vi "Get Cells (2D Row Part String).vi"(6 "Column":i32, 8 "error in (no error)":errorcluster, 9 "Row":i32, 10 "Sheet Reference":refnum<k24>) -> (0 "error out":errorcluster, 2 "Sheet Reference out":refnum<k24>, 5 "Values":string[][](array[string]))   [LabVIEW 2014]
doc: "Reads a row from the Sheet Reference. Row specifies which row to read from. Column specifies the starting column to read from (default of 0 for the full row)."
uses:
  C:/Users/LENOVO/Desktop/CodeSpace GUI/LVExcel/Resources/NPOI 2.1.1 dotnet2/NPOI.dll
  Resources/NPOI 2.1.1 dotnet2/NPOI.dll
  <vilib>/ErrorRing/Error Ring.xnode
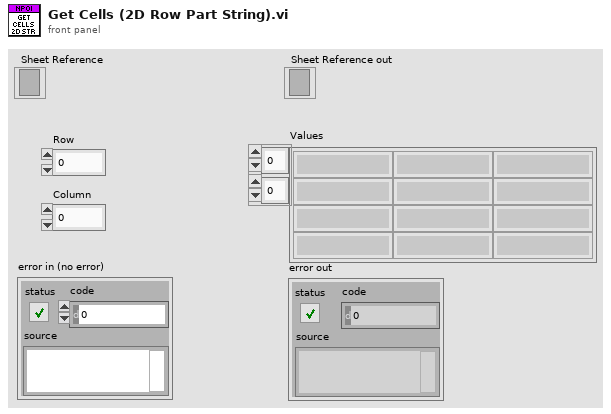
[diagram p1: front panel]
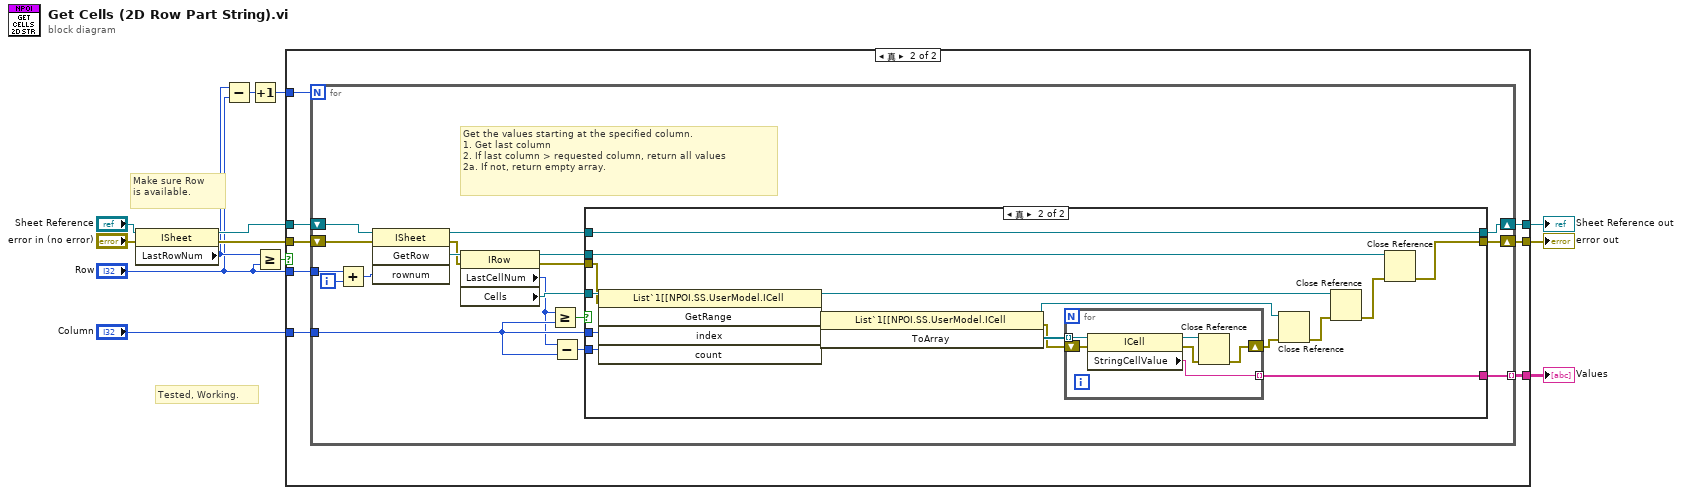
[diagram p0: block diagram]
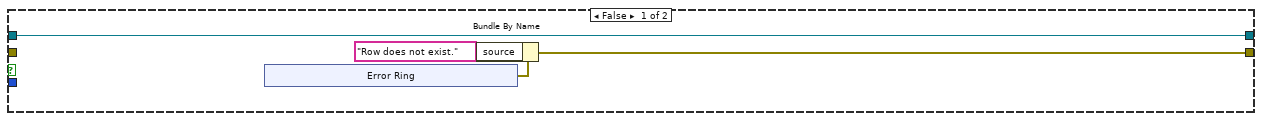
[diagram p2: hidden frame]
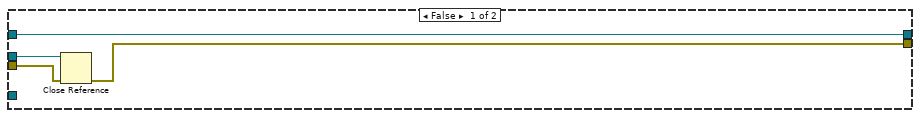
[diagram p3: hidden frame]
diagram:
  # "Tested, Working."
  # "Make sure Row\nis available."
  n1 = property class="ISheet"(reference="Sheet Reference", error in="error in (no error)") -> (reference out=w6:refnum<k24>, error out=w8:errorcluster, "LastRowNum"=w3:i32)
  n2 = Subtract(x=w3, y="Row") -> (x-y=w4:i32)
  n3 = Increment(x=w4) -> (x+1=w1:i32)
  n4 = Greater Or Equal?(x=w3, y="Row") -> (x >= y?=w5:bool)
  n5 = case shown="真" w5 {
    tunnel: w8 -> [_ w26]
    tunnel: w6 -> [w14 w25]
    tunnel: "Row" -> [_ w24]
    tunnel: [w14 w23] -> w13
    tunnel: [_ w22] -> w12
    tunnel: [w15 w21] -> w11
    tunnel: "Column" -> [_ w20]
    tunnel: w1 -> [_ w19]
    frame False {
      n6 = xnode "Error Ring"() -> ("错误输出"=w17:errorcluster)
      n7 = Bundle By Name(cluster=w17, "source"="Row does not exist.") -> (w15:errorcluster)
    }
    frame True {
      n8 = for {
        N: w19 -> [_]
        tunnel: w24 -> [w39]
        tunnel: [w37] -> w22 mode=indexing
        tunnel: w20 -> [w35]
        shift-right: [w38] -> w23
        shift-left: w25 -> [w40]
        shift-right: [w36] -> w21
        shift-left: w26 -> [w41]
        i -> [w27]
        # "Get the values starting at the specified column.\n1. Get last column\n2. If last column > requested column, return all values\n2a. If not, return empty array."
        n9 = Add(x=w39, y=w27) -> (x+y=w28:i32)
        n10 = invoke class="ISheet" method="GetRow"(reference=w40, error in=w41, "rownum"=w28) -> (reference out=w42:refnum<k24>, error out=w43:errorcluster, "GetRow"=w44:refnum<k24>)  [unwired: 1 in, 1 out]
        n11 = property class="IRow"(reference=w44, error in=w43) -> (reference out=w32:refnum<k24>, error out=w31:errorcluster, "LastCellNum"=w30:i16, "Cells"=w34:refnum<k24>)
        n12 = Greater Or Equal?(x=w30, y=w35) -> (x >= y?=w33:bool)
        n13 = Subtract(x=w30, y=w35) -> (x-y=w29:i32)
        n14 = case shown="真" w33 {
          tunnel: [_ w64] -> w37
          tunnel: w34 -> [_ w62]
          tunnel: w32 -> [w48 w54]
          tunnel: w31 -> [w47 w60]
          tunnel: [w46 w52] -> w36
          tunnel: w42 -> [w45 w51]
          tunnel: [w45 w51] -> w38
          tunnel: w35 -> [_ w50]
          tunnel: w29 -> [_ w49]
          frame False {
            n15 = Close Reference(reference=w48, error in (no error)=w47) -> (error out=w46:errorcluster)
          }
          frame True {
            n16 = invoke class="List`1[[NPOI.SS.UserModel.ICell" method="GetRange"(reference=w62, error in=w60, "index"=w50, "count"=w49) -> (reference out=w56:refnum<k24>, error out=w59:errorcluster, "GetRange"=w63:refnum<k24>)  [unwired: 1 in, 2 out]
            n17 = invoke class="List`1[[NPOI.SS.UserModel.ICell" method="ToArray"(reference=w63, error in=w59) -> (reference out=w58:refnum<k24>, error out=w61:errorcluster, "ToArray"=w65:refnum<k24>[])  [unwired: 1 in]
            n18 = for {
              tunnel: w65 -> [w71] mode=indexing
              tunnel: [w70] -> w64 mode=indexing
              shift-right: [w67] -> w57
              shift-left: w61 -> [w66]
              n19 = property class="ICell"(reference=w71, error in=w66) -> (reference out=w68:refnum<k24>, error out=w69:errorcluster, "StringCellValue"=w70:string)
              n20 = Close Reference(reference=w68, error in (no error)=w69) -> (error out=w67:errorcluster)
            }
            n21 = Close Reference(reference=w58, error in (no error)=w57) -> (error out=w55:errorcluster)
            n22 = Close Reference(reference=w56, error in (no error)=w55) -> (error out=w53:errorcluster)
            n23 = Close Reference(reference=w54, error in (no error)=w53) -> (error out=w52:errorcluster)
          }
        }
      }
    }
  }
  "Sheet Reference out" <- w13
  "error out" <- w11
  "Values" <- w12
